vi "Send Perform Action on Target.vi"(7 "Message Priority (Normal)":T1=enum."Normal", 8 "error in":errorcluster, 9 "Input":variant, 10 "Task-Point Ident":string, 11 "Message Enqueuer":refnum<class "Message Enqueuer.lvclass">) -> (0 "error out":errorcluster, 1 "Output":variant, 3 "Message Enqueuer out":refnum<class "Message Enqueuer.lvclass">)   [LabVIEW 2023, in "ISeries Actor.lvlib" / "Perform Action on Target Msg.lvclass"]
doc: "This VI sends the message to an actor."
uses:
  Perform Action on Target Msg.lvclass
  <vilib>/ActorFramework/Reply Msg/Reply Msg.lvclass
  <vilib>/ActorFramework/Message Enqueuer/Message Enqueuer.lvclass
  <vilib>/ActorFramework/Message Enqueuer/Message Priority.ctl
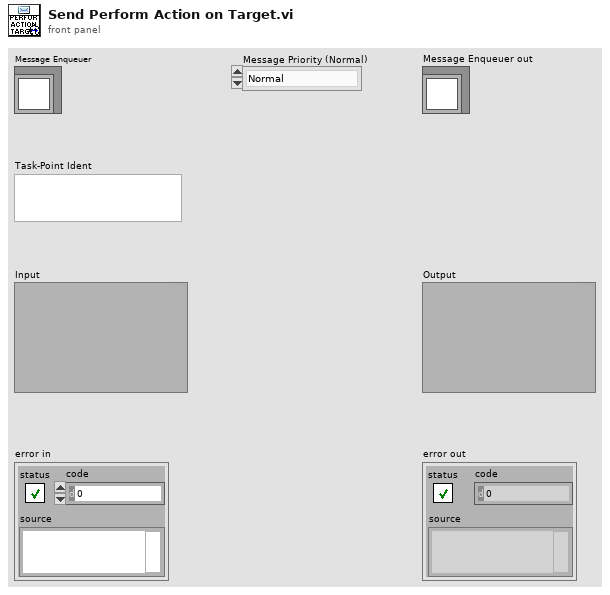
[diagram p1: front panel]
types:
  T1 = typedef "Actor Framework.lvlib/Message Enqueuer.lvclass/Message Priority.ctl" = enum16{"Low", "Normal", "High"}
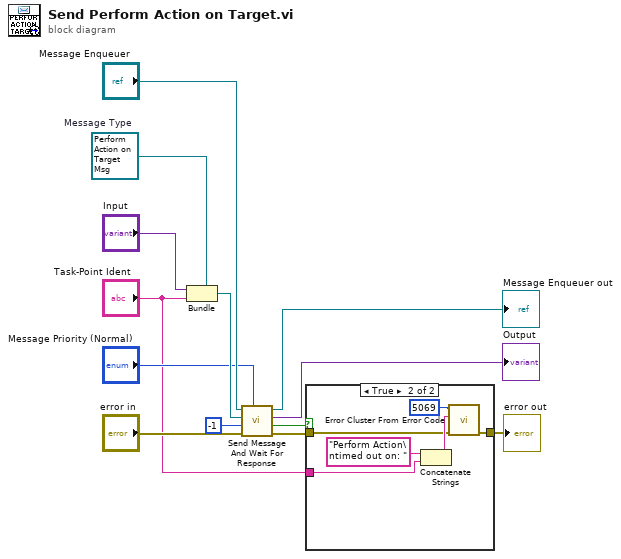
[diagram p0: block diagram]
diagram:
  w11 = refnum<class "Perform Action on Target Msg.lvclass"> refnum  # Message Type
  n1 = Bundle(cluster=w11, "Input", "Task-Point Ident") -> (w10:refnum<class "Perform Action on Target Msg.lvclass">)
  n2 = call <vilib>:"Send Message And Wait For Response.vi"("Message Priority (Normal)"="Message Priority (Normal)", "error in (no error)"="error in", "timeout in ms (-1)"=-1, "Original Message"=w10, "Message Enqueuer in"="Message Enqueuer") -> ("error out"=w5:errorcluster, "timed out?"=w4:bool, "Reply"=→"Output":variant, "Message Enqueuer out"=→"Message Enqueuer out":refnum<class "Message Enqueuer.lvclass">)  [unwired: 3 in]
  n3 = case shown="True" w4 {
    tunnel: w5 -> [w14 w16]
    tunnel: [w14 w20] -> w2
    tunnel: "Task-Point Ident" -> [_ w15]
    frame False {
    }
    frame True {
      n4 = Concatenate Strings("Perform Action\ntimed out on: ", w15) -> (w17:string)
      n5 = call <vilib>:"Error Cluster From Error Code.vi"("error in (no error)"=w16, "error message (\"\")"=w17, "error code (0)"=5069) -> ("error out"=w20:errorcluster)  [unwired: 6 in]
    }
  }
  "error out" <- w2
